vi "New File Log.vi"(4 "timestamp format (ISO8601)":string="%^<%Y-%m-%dT%H:%M:%S%3u>TZ", 6 "line format":string="{{timestamp}} | {{level}} | {{context}} | {{message}}", 7 "context":string, 8 "error in (no error)":errorcluster, 9 "write timeout (100ms)":i32=100, 10 "level":T1 items=["OFF"=0, "FATAL"=100, "ERROR"=200, "WARN"=300, "INFO"=400, "DEBUG"=500, "TRACE"=600, "ALL"=65535], 11 "Path":path) -> (0 "error out":errorcluster, 3 "File Log Provider out":refnum<data-value>)   [LabVIEW 2019, in "File Log Provider.lvclass"]
doc: "<b>Description</b> Create a new file logger with specified line and timestamp formats.\n\nBSD 3-Clause License\n\nCopyright (c) 2021, TauTerra, LLC\nAll rights reserved.\n\nRedistribution and use in source and binary forms, with or without\nmodification, are permitted provided that the following conditions are met:\n\n1. Redistributions of source code must retain the above copyright notice, this\n list of conditions and the following disclaimer.\n\n2. Redistributions in binary form must reproduce the above copyright notice,\n this list of conditions and the following disclaimer in the documentation\n and/or other materials provided with the distribution.\n\n3. Neither the name of the copyright holder nor the names of its\n contributors may be used to endorse or promote products derived from\n this software without specific prior written permission.\n\nTHIS SOFTWARE IS PROVIDED BY THE COPYRIGHT HOLDERS AND CONTRIBUTORS \"AS IS\"\nAND ANY EXPRESS OR IMPLIED WARRANTIES, INCLUDING, BUT NOT LIMITED TO, THE\nIMPLIED WARRANTIES OF MERCHANTABILITY AND FITNESS FOR A PARTICULAR PURPOSE ARE\nDISCLAIMED. IN NO EVENT SHALL THE COPYRIGHT HOLDER OR CONTRIBUTORS BE LIABLE\nFOR ANY DIRECT, INDIRECT, INCIDENTAL, SPECIAL, EXEMPLARY, OR CONSEQUENTIAL\nDAMAGES (INCLUDING, BUT NOT LIMITED TO, PROCUREMENT OF SUBSTITUTE GOODS OR\nSERVICES; LOSS OF USE, DATA, OR PROFITS; OR BUSINESS INTERRUPTION) HOWEVER\nCAUSED AND ON ANY THEORY OF LIABILITY, WHETHER IN CONTRACT, STRICT LIABILITY,\nOR TORT (INCLUDING NEGLIGENCE OR OTHERWISE) ARISING IN ANY WAY OUT OF THE USE\nOF THIS SOFTWARE, EVEN IF ADVISED OF THE POSSIBILITY OF SUCH DAMAGE."
uses:
  File Log Provider.lvclass
  Log Service/public/level.ctl
  File Log Provider.lvclass/File Log Provider.ctl
  206e80bf-bc4f-4e86-b2bc-2fb61efe7177.vi
  subVIs/monitor_log_queue.vi
  Queue Log Provider/Queue Log Provider.lvclass
  Log Service/Log Service.lvclass
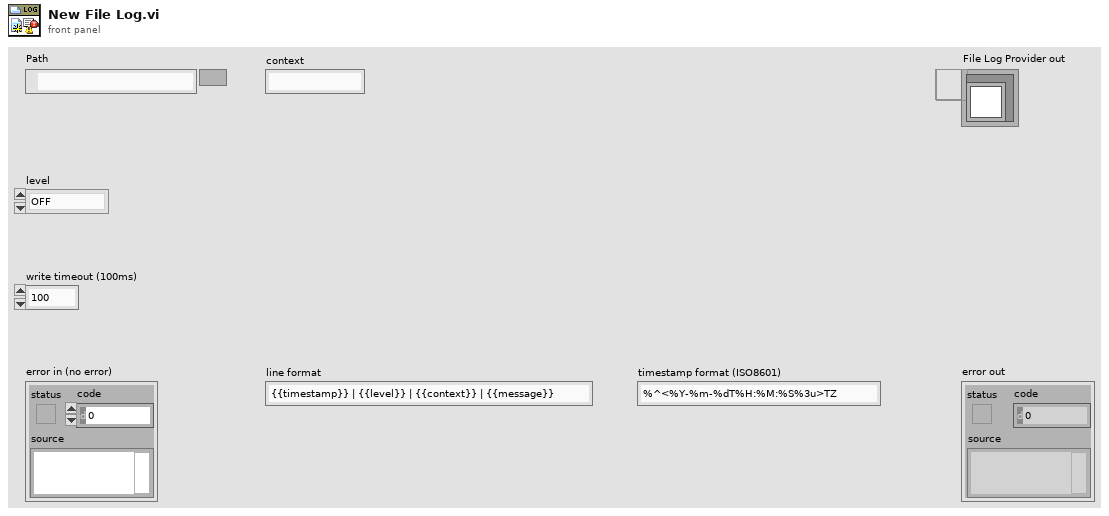
[diagram p1: front panel]
types:
  T1 = typedef "Utility API.lvlib/Log Service.lvclass/level.ctl" = u16
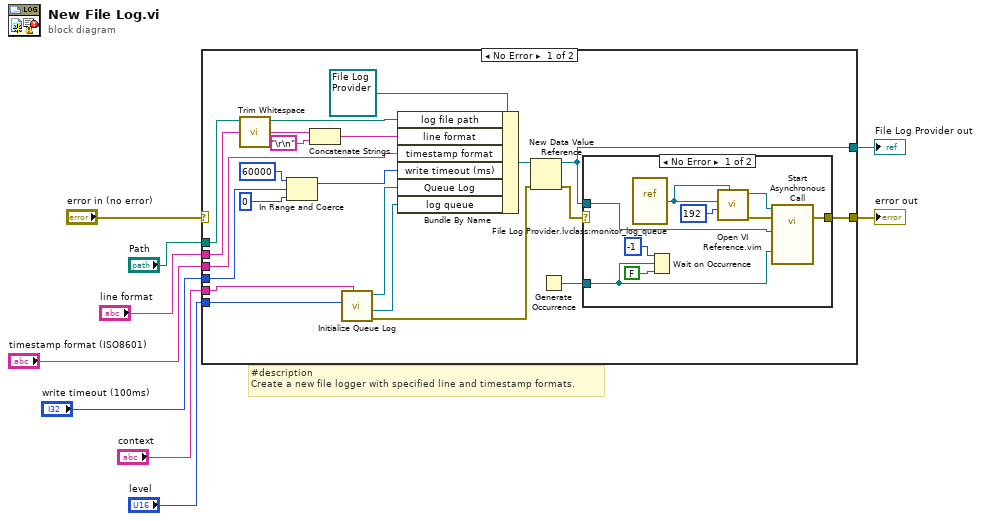
[diagram p0: block diagram]
diagram:
  # "#description\nCreate a new file logger with specified line and timestamp formats."
  n1 = case shown="No Error" "error in (no error)" {
    selector: "error in (no error)" -> [_ w41]
    tunnel: [w21 w41] -> w8
    tunnel: [w22 _] -> w7
    tunnel: "Path" -> [w29 _]
    tunnel: "level" -> [w18 _]
    tunnel: "context" -> [w27 _]
    tunnel: "line format" -> [w28 _]
    tunnel: "write timeout (100ms)" -> [w17 _]
    tunnel: "timestamp format (ISO8601)" -> [w14 _]
    frame No Error {
      n2 = call <vilib>:"Trim Whitespace.vi"("string"=w28) -> ("trimmed string"=w13:string)  [unwired: 1 in]
      n3 = In Range and Coerce(upper limit=60000, x=w17, lower limit=0) -> (coerced(x)=w15:i32)  [unwired: 1 out]
      n4 = Concatenate Strings(w13, "\r\n") -> (w12:string)
      n5 = call "Initialize Queue Log.vi"("context"=w27, "level"=w18) -> ("error out"=w24:errorcluster, "queue out"=w20:refnum<queue>, "Queue Log Provider out"=w26:refnum<class "Queue Log Provider.lvclass">)  [unwired: 7 in]
      n6 = Bundle By Name(cluster=refnum<class "File Log Provider.lvclass"> refnum ("File Log Provider in"), "log file path"=w29, "line format"=w12, "timestamp format"=w14, "write timeout (ms)"=w15, "Queue Log"=w26, "log queue"=w20) -> (w30:refnum<class "File Log Provider.lvclass">)
      n7 = New Data Value Reference(data value=w30, error in=w24) -> (data value reference=w22:refnum<data-value>, error out=w23:errorcluster)
      n8 = Generate Occurrence() -> (w10:refnum<k4>)
      n9 = case shown="No Error" w23 {
        selector: w23 -> [_ w40]
        tunnel: w22 -> [w36 _]
        tunnel: [w34 w40] -> w21
        tunnel: w10 -> [w31 _]
        frame No Error {
          n10 = vi-ref "File Log Provider.lvclass:monitor_log_queue.vi"() -> (w39:refnum<vi>)
          n11 = Wait on Occurrence(1:FALSE ("ignore previous (T)"), 2:w31, 3:-1 ("ms timeout (-1)")) -> ()  [unwired: 1 out]
          n12 = call "Open VI Reference.vim"("type specifier VI Refnum (for type only)"=w39, "options"=192, "vi reference"=w39) -> ("error out"=w35:errorcluster, "vi reference out"=w37:refnum<vi>)  [unwired: 7 in]
          n13 = call-by-ref "Start Asynchronous Call"(reference=w37, error in=w35, "occurrence"=w31, "File Log Provider in"=w36) -> (error out=w34:errorcluster)  [unwired: 10 in, 1 out]
        }
        frame Error {
        }
      }
    }
    frame Error {
    }
  }
  "error out" <- w8
  "File Log Provider out" <- w7
